vi "Send Actual Record Length.vi"(7 "Message Priority (Normal)":T1=enum."Normal", 8 "error in (no error)":errorcluster, 11 "Message Enqueuer":refnum<class "Message Enqueuer.lvclass">) -> (0 "error out":errorcluster, 3 "Message Enqueuer out":refnum<class "Message Enqueuer.lvclass">)   [LabVIEW 2014, in "CS++Scope.lvlib" / "Actual Record Length Msg.lvclass"]
doc: "Sends the <B>CS++Scope.lvlib:Actual Record Length Msg.lvclass</B> message.\n\n<B>CS++Scope.lvlib:CS++Scope.lvclass:Actual Record Length.vi</B> Description:\n\nThis VI returns the actual number of points the oscilloscope acquires for each channel. After you configure the oscilloscope for an acquisition, call this VI to determine the size of the waveforms that the oscilloscope acquires. The value is greater than or equal to the minimum number of points you specify in the IviScope Configure Acquisition Record VI. \nYou can use this value as the Waveform Size parameter of the IviScope Read Waveform and IviScope Fetch Waveform VIs."
uses:
  Actual Record Length Msg.lvclass
  <vilib>/ActorFramework/Message Enqueuer/Message Enqueuer.lvclass
  <vilib>/ActorFramework/Message Enqueuer/Message Priority.ctl
  <vilib>/ActorFramework/Message/Message.lvclass
  <vilib>/ActorFramework/Message Enqueuer/Message Enqueuer.lvclass/Message Enqueuer.ctl
  <vilib>/ActorFramework/Message Priority Queue/Priority Enqueue.vi
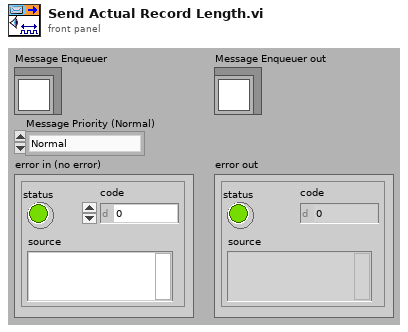
[diagram p1: front panel]
types:
  T1 = typedef "Actor Framework.lvlib/Message Enqueuer.lvclass/Message Priority.ctl" = enum16{"Low", "Normal", "High"}
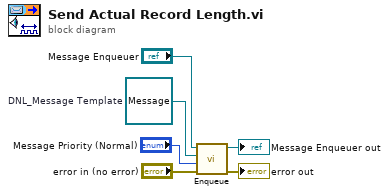
[diagram p0: block diagram]
diagram:
  w1 = refnum<class "Message.lvclass"> refnum  # DNL_Message Template
  n1 = call <vilib>:"Enqueue.vi"("error in (no error)"="error in (no error)", "Message Priority (Normal)"="Message Priority (Normal)", "Message"=w1, "Message Enqueuer in"="Message Enqueuer") -> ("error out"=→"error out":errorcluster, "Message Enqueuer out"=→"Message Enqueuer out":refnum<class "Message Enqueuer.lvclass">)  [unwired: 6 in]
